vi "1. EncoderTest.vi"(8 "error in (no error)":errorcluster, 10 "Reset Counter":bool, 11 "stop":bool) -> (0 "error out":errorcluster, 1 "StickEncoder (deg)":dbl, 2 "MotorEncoder (deg)":dbl)   [LabVIEW 2019, in "SJCube.lvlib"]
uses:
  SJCube.lvlib
panel:
  # "ATTENTION:\n\nClick the T/F contant on both ENC VIs, make sure the directions are the same as the figures below."
  # "StickEncoder"
  # "MotorEncoder"
  # "deg 60"
  # "deg -45"
  # "deg 0"
  # "deg 45"
  # "deg -30"
  # "deg 0"
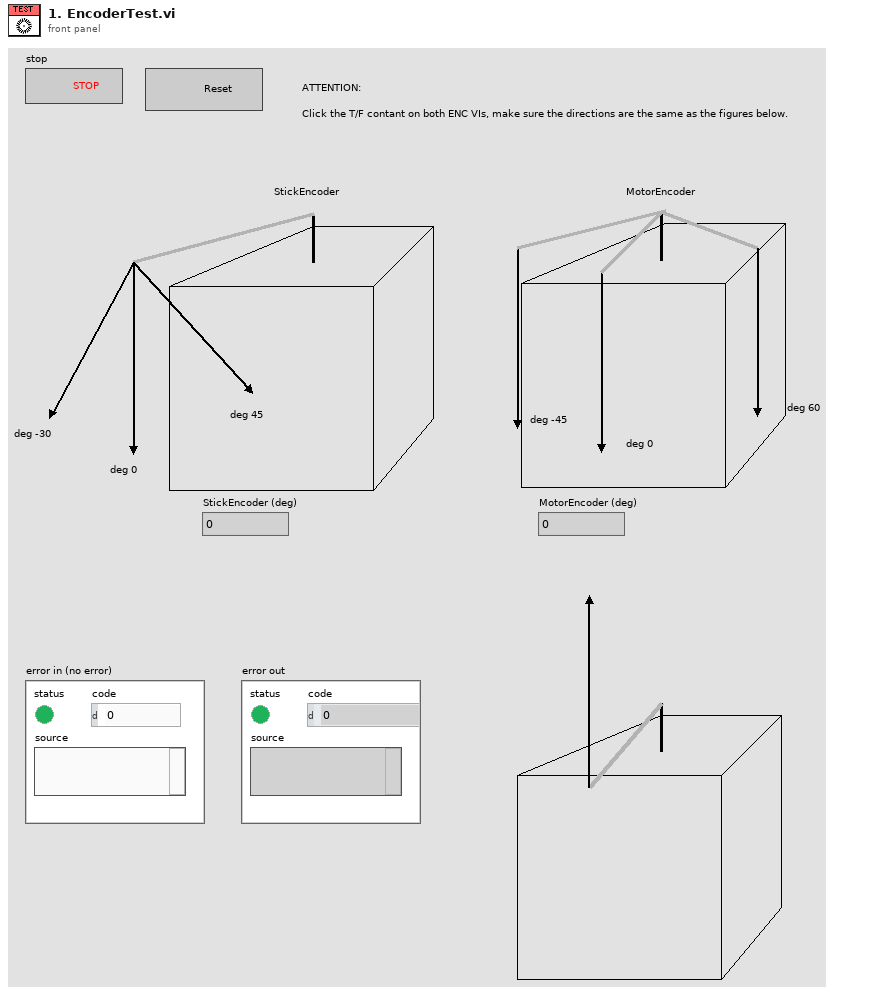
[diagram p1: front panel]
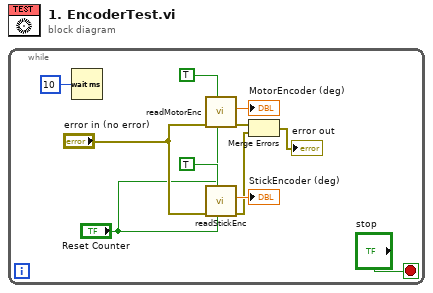
[diagram p0: block diagram]
diagram:
  n1 = while {
    stop <- "stop" stop-if-true
    n2 = Wait (ms)(milliseconds to wait=u32 10) -> ()  [unwired: 1 out]
    n3 = call "readMotorEnc.vi"("Reset Counter"="Reset Counter", "Reverse ENC?"=TRUE, "error in (no error)"="error in (no error)") -> ("error out"=w3:errorcluster, "MotorEncoder (deg)"=→"MotorEncoder (deg)":dbl)  [unwired: 7 in]
    n4 = call "readStickEnc.vi"("Reset Counter"="Reset Counter", "Reverse ENC?"=TRUE, "error in (no error)"="error in (no error)") -> ("error out"=w4:errorcluster, "StickEncoder (deg)"=→"StickEncoder (deg)":dbl)  [unwired: 7 in]
    n5 = Merge Errors(w3, w4) -> (→"error out":errorcluster)
  }
